vi "Classify.vi"(9 "Array 3":string[](array[string]), 10 "delimiters":string[](array[string]), 11 "Array in":string[](array[string])) -> (2 "Array out":string[](array[string]), 3 "Array 4":T1(array[ring]))   [LabVIEW 2015]
uses:
  <vilib>/regexp/Match Regular Expression.xnode
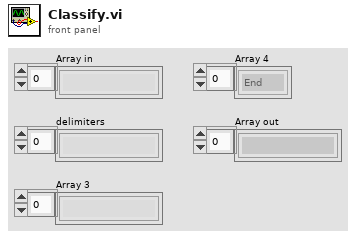
[diagram p1: front panel]
types:
  T1 = enum16{"End", "Boolean", "Named Cluster", "Unnamed Cluster", "Array", "String", "Decimal", "FloatingPoint", "End Array", "End Cluster"}[]
  T2 = enum16{"End", "Boolean", "Named Cluster", "Unnamed Cluster", "Array", "String", "Decimal", "FloatingPoint", "End Array", "End Cluster"}
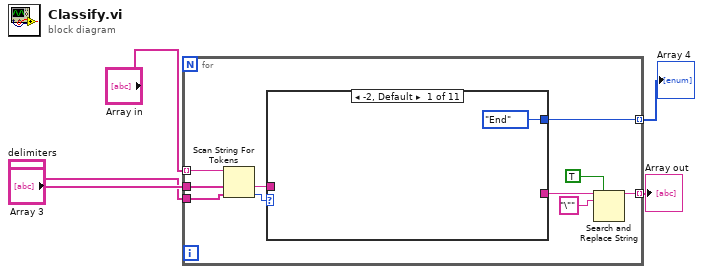
[diagram p0: block diagram]
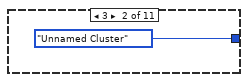
[diagram p2: hidden frame]
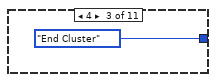
[diagram p3: hidden frame]
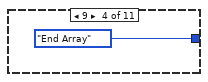
[diagram p4: hidden frame]
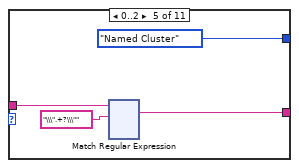
[diagram p5: hidden frame]
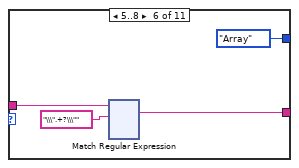
[diagram p6: hidden frame]
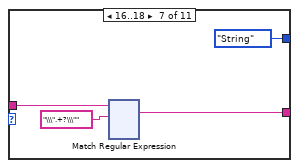
[diagram p7: hidden frame]
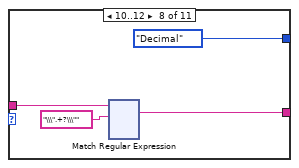
[diagram p8: hidden frame]
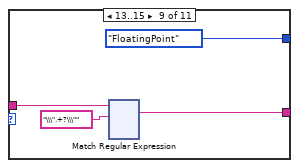
[diagram p9: hidden frame]
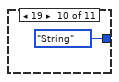
[diagram p10: hidden frame]
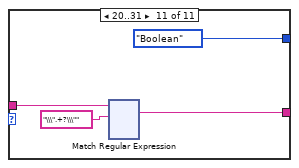
[diagram p11: hidden frame]
diagram:
  n1 = for {
    tunnel: "Array in" -> [w15] mode=indexing
    tunnel: "delimiters" -> [w14]
    tunnel: "Array 3" -> [w13]
    tunnel: [w11] -> w2 mode=indexing
    tunnel: [w8] -> w4 mode=indexing
    n2 = Scan String For Tokens(6:w14, 7:w13, 9:w15) -> (0:w12:i32, 1:w10:string)  [unwired: 3 in, 2 out]
    n3 = case shown="-2, Default" w12 {
      tunnel: [T2."End" T2."Unnamed Cluster" T2."End Cluster" T2."End Array" T2."Named Cluster" T2."Array" T2."String" T2."Decimal" T2."FloatingPoint" T2."String" T2."Boolean"] -> w11
      tunnel: w10 -> [_ _ _ _ w21 w139 w257 w375 w493 _ w612]
      tunnel: [_ _ _ _ w20 w138 w256 w374 w492 _ w611] -> w9
      frame -2, Default {
      }
      frame 3 {
      }
      frame 4 {
      }
      frame 9 {
      }
      frame 0..2 {
        n4 = xnode "Match Regular Expression"("input string"=w21, "regular expression"="\\\".+?\\\"") -> ("whole match"=w20:string)  [unwired: 4 in, 4 out]
      }
      frame 5..8 {
        n5 = xnode "Match Regular Expression"("input string"=w139, "regular expression"="\\\".+?\\\"") -> ("whole match"=w138:string)  [unwired: 4 in, 4 out]
      }
      frame 16..18 {
        n6 = xnode "Match Regular Expression"("input string"=w257, "regular expression"="\\\".+?\\\"") -> ("whole match"=w256:string)  [unwired: 4 in, 4 out]
      }
      frame 10..12 {
        n7 = xnode "Match Regular Expression"("input string"=w375, "regular expression"="\\\".+?\\\"") -> ("whole match"=w374:string)  [unwired: 4 in, 4 out]
      }
      frame 13..15 {
        n8 = xnode "Match Regular Expression"("input string"=w493, "regular expression"="\\\".+?\\\"") -> ("whole match"=w492:string)  [unwired: 4 in, 4 out]
      }
      frame 19 {
      }
      frame 20..31 {
        n9 = xnode "Match Regular Expression"("input string"=w612, "regular expression"="\\\".+?\\\"") -> ("whole match"=w611:string)  [unwired: 4 in, 4 out]
      }
    }
    n10 = Search and Replace String(replace all?=TRUE ("replace all? (F)"), input string=w9, search string="\"") -> (result string=w8:string)  [unwired: 5 in, 3 out]
  }
  "Array out" <- w4
  "Array 4" <- w2
